vi "Image Cap Get SAED Sensitivity.vi"(8 "error in (no error)":errorcluster, 10 "nSens":i32, 11 "nSensorIP":u32) -> (0 "error out":errorcluster, 2 "nSens out":i32, 3 "function return":i32)   [LabVIEW 2017, in "BonTechDetector.lvlib"]
doc: "DLLFunction int __stdcall ImageCapGetSAEDSensitivity(unsigned int nSensorIP, int* nSens);"
uses:
  BonTechDetector.lvlib
  lib/ImageCaptureDLL.dll
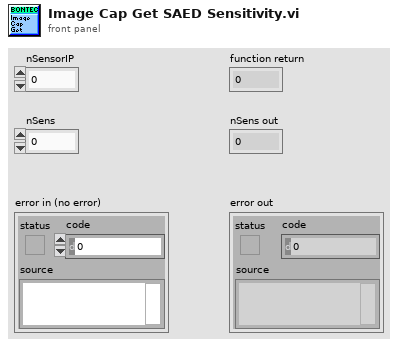
[diagram p1: front panel]
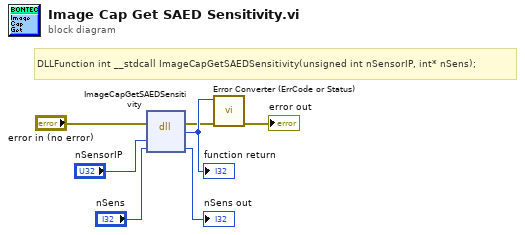
[diagram p0: block diagram]
diagram:
  # "DLLFunction int __stdcall ImageCapGetSAEDSensitivity(unsigned int nSensorIP, int* nSens);"
  n1 = dll-call lib="F:/BonTechFlatPanelLVDriver/lib/ImageCaptureDLL.*" fn="ImageCapGetSAEDSensitivity"(error in="error in (no error)", "nSensorIP"="nSensorIP", "nSens"="nSens") -> (error out=w2:errorcluster, w7:i32, "nSens"=→"nSens out":i32)  [unwired: 3 in, 1 out]
  "function return" <- w7
  n2 = call "Error Converter (ErrCode or Status).vi"("error in (no error)"=w2, "error code"=w7) -> ("error out"=→"error out":errorcluster)  [unwired: 9 in]
